vi "SRV_Generate User Exit Event.vi"(8 "error in (no error)":errorcluster, 11 "User Exit Event":refnum<user-event>) -> (0 "error out":errorcluster, 3 "User Exit Event out":refnum<user-event>)   [LabVIEW 2014]
doc: "Broadcast the User Exit event to all event structures that are registered to handle the event.\n\n\nAuthor: Mike Schultz\n\n\nLogicPD, Inc\nwww.logicpd.com"
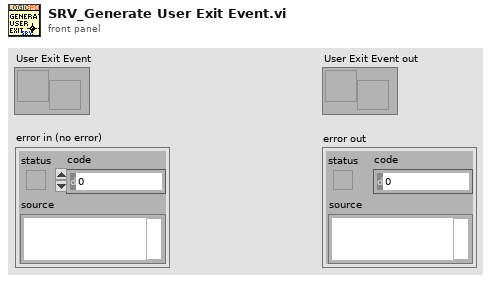
[diagram p1: front panel]
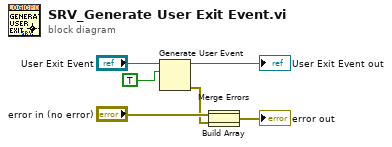
[diagram p0: block diagram]
diagram:
  n1 = Generate User Event(user event="User Exit Event", event data cluster=TRUE ("User Exit")) -> (user event out=→"User Exit Event out":refnum<user-event>, error out=w2:errorcluster)  [unwired: 2 in]
  n2 = Build Array("error in (no error)", w2) -> (w1:errorcluster[])
  n3 = Merge Errors(w1) -> (→"error out":errorcluster)
